vi "Read TriggerModulo.vi"(8 "error in (no error)":errorcluster, 11 "BME_DG_G05_Chnl in":refnum<class "BME_DG_G05P2_Chnl.lvclass">) -> (0 "error out":errorcluster, 2 "TriggerModulo":i32, 3 "BME_DG_G05_Chnl out":refnum<class "BME_DG_G05P2_Chnl.lvclass">)   [LabVIEW 2009, in "BME_DG_G05P2_Chnl.lvclass"]
uses:
  BME_DG_G05P2_Chnl.lvclass
  BME_DG_G05P2_Chnl.lvclass/BME_DG_G05P2_Chnl.ctl
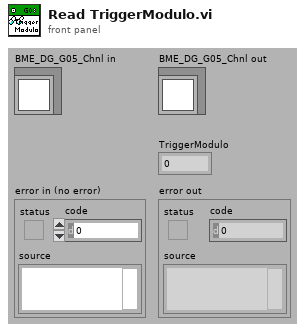
[diagram p1: front panel]
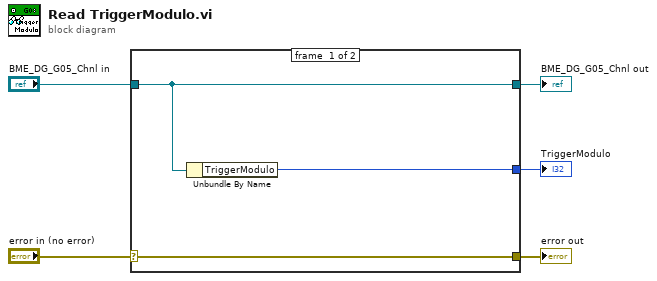
[diagram p0: block diagram]
diagram:
  n1 = case shown="No Error" "error in (no error)" {
    selector: "error in (no error)" -> [w8 w9]
    tunnel: [w8 w9] -> w4
    tunnel: [w7 w10] -> w2
    tunnel: "BME_DG_G05_Chnl in" -> [w7 w10]
    tunnel: [w6 _] -> w1
    frame #0 {
      n2 = Unbundle By Name(w7) -> ("TriggerModulo"=w6:i32)
    }
    frame #1 {
    }
  }
  "error out" <- w4
  "BME_DG_G05_Chnl out" <- w2
  "TriggerModulo" <- w1
